vi "Simple UDP Test.vi"() -> ()   [LabVIEW 2016, in "instr.lvlib"]
doc: "Test VI using all other VIs.\nThis should help you to gest startet with your application."
uses:
  instr.lvlib
  IO State.ctl
  Digital Mode.ctl
panel:
  in  "local port":u16=61557
  in  "controllino ip":string="192.168.0.12"
  in  "controllino port":u16=8888
  in  "Send RAW":bool
  out "Memory Data Readback":i16
  in  "Memory Value":i16
  in  "Memory Addr":u16
  in  "Set Memory":bool
  in  "Set All Config":bool
  out "Digital Mode":T1[](array[typedef]) items=["Output"=79, "Input_Pullup"=80, "Input"=73]
  out "Inputs":bool[](array[boolean])
  out "dt (ms)":u32
  out "Analog Value":u16
  in  "Read Analog":bool
  out "Analog Values":u16[](array[numeric])
  in  "Analog Number":u16
  in  "Digital Mode":T1=73 items=["Output"=79, "Input_Pullup"=80, "Input"=73]
  in  "Set Config":bool
  in  "Set All Relay":bool
  in  "Set All Digital":bool
  in  "Digital State":T2 items=["LOW", "HIGH"]
  in  "Digital Number":u16
  in  "Relay State":T2 items=["LOW", "HIGH"]
  in  "Relay Number":u16
  in  "Set Digital":bool
  in  "Set Relay":bool
  out "Digitals":bool[](array[boolean])
  out "Relays":bool[](array[boolean])
  in  "stop":bool
  out "RAW Reply":string
  in  "RAW":string
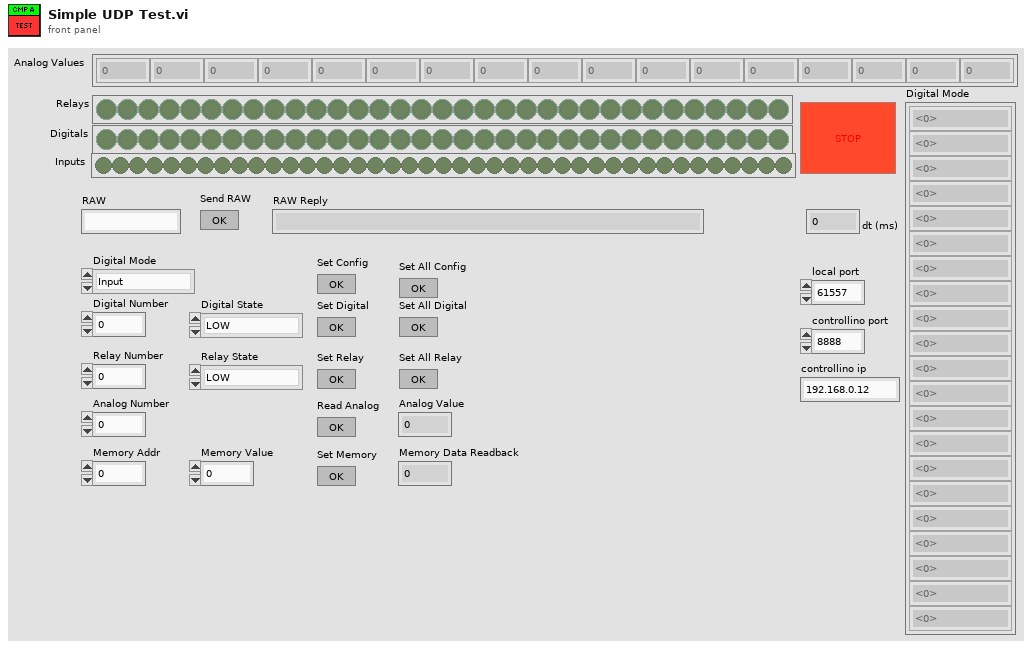
[diagram p1: front panel]
types:
  T1 = typedef "instr.lvlib/Digital Mode.ctl" = u16
  T2 = typedef "instr.lvlib/IO State.ctl" = u16
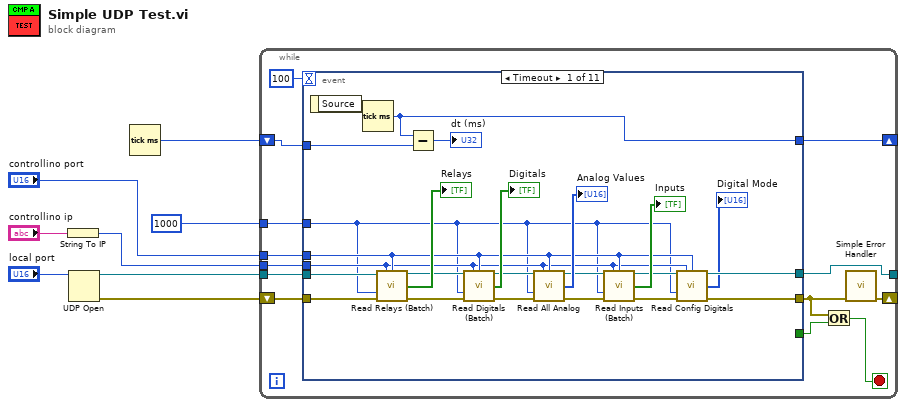
[diagram p0: block diagram]
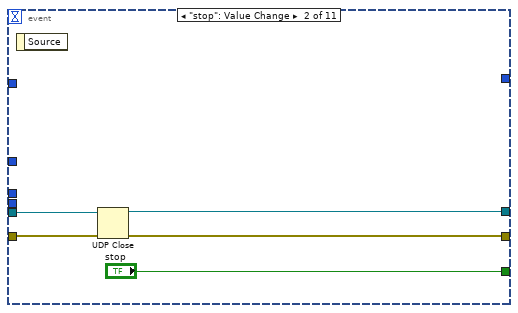
[diagram p2: hidden frame]
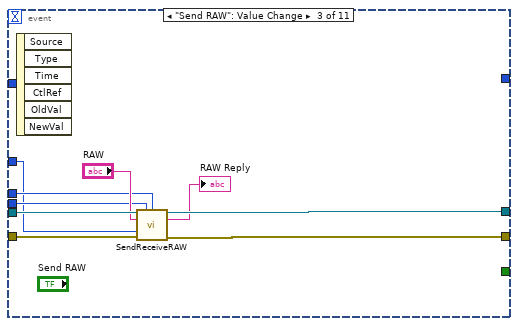
[diagram p3: hidden frame]
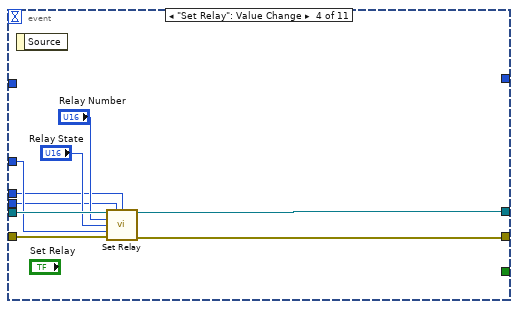
[diagram p4: hidden frame]
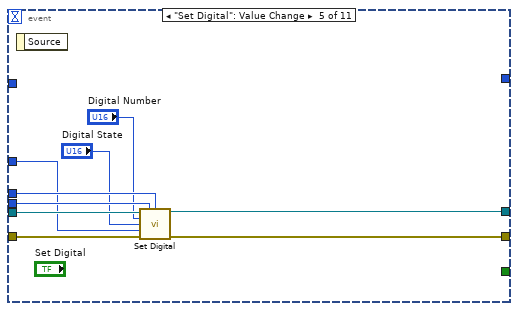
[diagram p5: hidden frame]
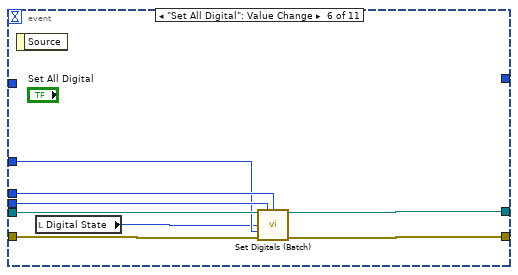
[diagram p6: hidden frame]
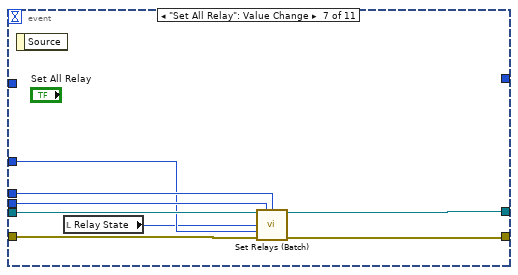
[diagram p7: hidden frame]
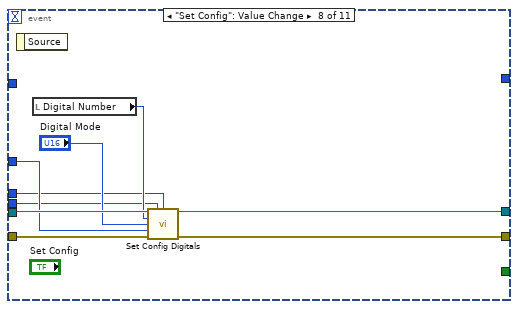
[diagram p8: hidden frame]
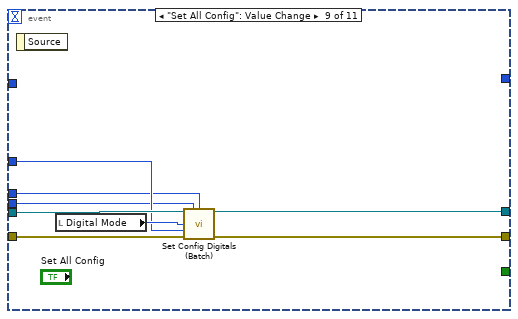
[diagram p9: hidden frame]
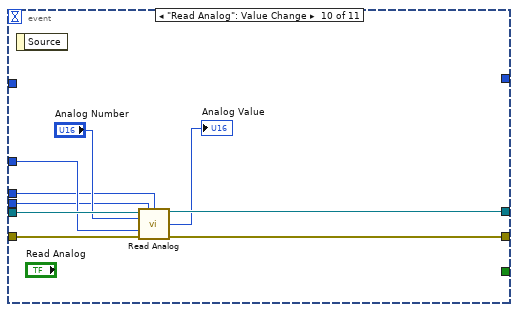
[diagram p10: hidden frame]
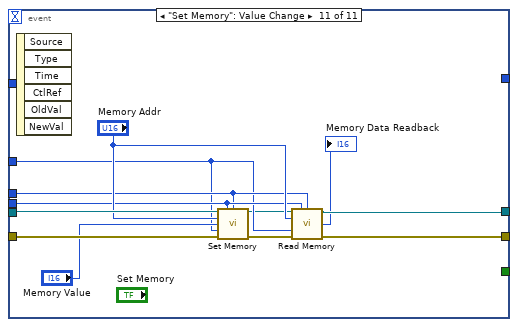
[diagram p11: hidden frame]
diagram:
  n1 = String To IP(1:"controllino ip") -> (0:w4:u32)
  n2 = UDP Open(11:"local port") -> (port=w6:refnum<k16>, 0:w5:errorcluster)  [unwired: 4 in, 1 out]
  n3 = Tick Count (ms)() -> (millisecond timer value=w1:u32)
  n4 = while {
    tunnel: w6 -> [w20]
    tunnel: [w18] -> _
    tunnel: w4 -> [w17]
    tunnel: "controllino port" -> [w16]
    tunnel: 1000 ("timeout ms (1000)") -> [w15]
    shift-right: [w14] -> _
    shift-left: w5 -> [w19]
    shift-right: [w12] -> _
    shift-left: w1 -> [w13]
    stop <- w9 stop-if-true
    n5 = event shown="[0] Timeout" {
      selector: _ -> [_ _ _ _ _ _ _ _ _ _ _]
      dyn-events: _ -> [_ _ _ _ _ _ _ _ _ _ _]
      timeout: 100 -> [_ _ _ _ _ _ _ _ _ _ _]
      tunnel: w20 -> [w44 w47 w54 w66 w74 w81 w92 w98 w107 w117 w129]
      tunnel: w19 -> [w43 w48 w58 w67 w76 w84 w91 w101 w108 w118 w130]
      tunnel: [w28 w46 w57 w64 w75 w83 w90 w100 w102 w112 w127] -> w11
      tunnel: [w27 w45 w56 w65 w73 w82 w89 w99 w103 w111 w121] -> w18
      tunnel: w17 -> [w24 _ w52 w60 w72 w79 w87 w93 w105 w113 w124]
      tunnel: w16 -> [w25 _ w51 w59 w71 w80 w88 w94 w104 w114 w123]
      tunnel: w15 -> [w23 _ w50 w62 w68 w78 w86 w95 w106 w115 w122]
      tunnel: [_ "stop" _ _ _ _ _ _ _ _ _] -> w10
      tunnel: w13 -> [w35 _ _ _ _ _ _ _ _ _ _]
      tunnel: [w34 _ _ _ _ _ _ _ _ _ _] -> w12
      event Timeout {
        n6 = event-data() -> ()  [unwired: 1 in, 1 out]
        n7 = Tick Count (ms)() -> (millisecond timer value=w34:u32)
        n8 = call "Read Relays (Batch).vi"("connection ID"=w44, "address"=w24, "port"=w25, "timeout ms (1000)"=w23, "error in (no error)"=w43) -> ("connection ID out"=w40:refnum<k16>, "Relays"=→"Relays":bool[], "error out"=w41:errorcluster)  [unwired: 7 in, 1 out]
        n9 = Subtract(x=w34, y=w35) -> (x-y=→"dt (ms)":u32)
        n10 = call "Read Digitals (Batch).vi"("connection ID"=w40, "address"=w24, "port"=w25, "timeout ms (1000)"=w23, "error in (no error)"=w41) -> ("connection ID out"=w38:refnum<k16>, "Digitals"=→"Digitals":bool[], "error out"=w37:errorcluster)  [unwired: 7 in, 1 out]
        n11 = call "Read All Analog.vi"("connection ID"=w38, "address"=w24, "port"=w25, "timeout ms (1000)"=w23, "error in (no error)"=w37) -> ("connection ID out"=w31:refnum<k16>, "Analog Values"=→"Analog Values":u16[], "error out"=w32:errorcluster)  [unwired: 7 in, 1 out]
        n12 = call "Read Inputs (Batch).vi"("connection ID"=w31, "address"=w24, "port"=w25, "timeout ms (1000)"=w23, "error in (no error)"=w32) -> ("connection ID out"=w26:refnum<k16>, "Inputs"=→"Inputs":bool[], "error out"=w29:errorcluster)  [unwired: 7 in, 1 out]
        n13 = call "Read Config Digitals.vi"("connection ID"=w26, "address"=w24, "port"=w25, "timeout ms (1000)"=w23, "error in (no error)"=w29) -> ("connection ID out"=w27:refnum<k16>, "Digital Mode"=→"Digital Mode":T1[], "error out"=w28:errorcluster)  [unwired: 7 in, 1 out]
      }
      event "stop": Value Change {
        n14 = event-data() -> ()  [unwired: 1 in, 1 out]
        n15 = UDP Close(connection ID=w47, 8:w48) -> (connection ID out=w45:refnum<k16>, error out=w46:errorcluster)
      }
      event "Send RAW": Value Change {
        n16 = event-data() -> ()  [unwired: 1 in, 6 out]
        n17 = call "SendReceiveRAW.vi"("connection ID"=w54, "address"=w52, "port"=w51, "RAW data in"="RAW", "timeout ms (1000)"=w50, "error in (no error)"=w58) -> ("connection ID out"=w56:refnum<k16>, "received data"=→"RAW Reply":string, "error out"=w57:errorcluster)  [unwired: 7 in]
      }
      event "Set Relay": Value Change {
        n18 = event-data() -> ()  [unwired: 1 in, 1 out]
        n19 = call "Set Relay.vi"("connection ID"=w66, "address"=w60, "port"=w59, "Relay Number"="Relay Number", "Relay State"="Relay State", "timeout ms (1000)"=w62, "error in (no error)"=w67) -> ("connection ID out"=w65:refnum<k16>, "error out"=w64:errorcluster)  [unwired: 6 in, 1 out]
      }
      event "Set Digital": Value Change {
        n20 = event-data() -> ()  [unwired: 1 in, 1 out]
        n21 = call "Set Digital.vi"("connection ID"=w74, "address"=w72, "port"=w71, "Digital Number"="Digital Number", "Digital State"="Digital State", "timeout ms (1000)"=w68, "error in (no error)"=w76) -> ("connection ID out"=w73:refnum<k16>, "error out"=w75:errorcluster)  [unwired: 6 in, 1 out]
      }
      event "Set All Digital": Value Change {
        n22 = event-data() -> ()  [unwired: 1 in, 1 out]
        n23 = local read "Digital State"() -> (w77:T2)
        n24 = call "Set Digitals (Batch).vi"("connection ID"=w81, "address"=w79, "port"=w80, "Digital State"=w77, "timeout ms (1000)"=w78, "error in (no error)"=w84) -> ("connection ID out"=w82:refnum<k16>, "error out"=w83:errorcluster)  [unwired: 7 in, 1 out]
      }
      event "Set All Relay": Value Change {
        n25 = event-data() -> ()  [unwired: 1 in, 1 out]
        n26 = local read "Relay State"() -> (w85:T2)
        n27 = call "Set Relays (Batch).vi"("connection ID"=w92, "address"=w87, "port"=w88, "Relay State"=w85, "timeout ms (1000)"=w86, "error in (no error)"=w91) -> ("connection ID out"=w89:refnum<k16>, "error out"=w90:errorcluster)  [unwired: 7 in, 1 out]
      }
      event "Set Config": Value Change {
        n28 = event-data() -> ()  [unwired: 1 in, 1 out]
        n29 = local read "Digital Number"() -> (w97:u16)
        n30 = call "Set Config Digitals.vi"("connection ID"=w98, "address"=w93, "port"=w94, "Digital Number"=w97, "Digital Mode"="Digital Mode", "timeout ms (1000)"=w95, "error in (no error)"=w101) -> ("connection ID out"=w99:refnum<k16>, "error out"=w100:errorcluster)  [unwired: 6 in, 1 out]
      }
      event "Set All Config": Value Change {
        n31 = event-data() -> ()  [unwired: 1 in, 1 out]
        n32 = local read "Digital Mode"() -> (w109:T1)
        n33 = call "Set Config Digitals (Batch).vi"("connection ID"=w107, "address"=w105, "port"=w104, "Digital Mode"=w109, "timeout ms (1000)"=w106, "error in (no error)"=w108) -> ("connection ID out"=w103:refnum<k16>, "error out"=w102:errorcluster)  [unwired: 7 in, 1 out]
      }
      event "Read Analog": Value Change {
        n34 = event-data() -> ()  [unwired: 1 in, 1 out]
        n35 = call "Read Analog.vi"("connection ID"=w117, "address"=w113, "port"=w114, "Analog Number"="Analog Number", "timeout ms (1000)"=w115, "error in (no error)"=w118) -> ("connection ID out"=w111:refnum<k16>, "Analog Value"=→"Analog Value":u16, "error out"=w112:errorcluster)  [unwired: 6 in, 1 out]
      }
      event "Set Memory": Value Change {
        n36 = event-data() -> ()  [unwired: 1 in, 6 out]
        n37 = call "Set Memory.vi"("connection ID"=w129, "address"=w124, "port"=w123, "Digital Number"="Memory Addr", "Data"="Memory Value", "timeout ms (1000)"=w122, "error in (no error)"=w130) -> ("connection ID out"=w119:refnum<k16>, "error out"=w126:errorcluster)  [unwired: 6 in, 1 out]
        n38 = call "Read Memory.vi"("connection ID"=w119, "address"=w124, "port"=w123, "Memory Address"="Memory Addr", "timeout ms (1000)"=w122, "error in (no error)"=w126) -> ("connection ID out"=w121:refnum<k16>, "Memory Data"=→"Memory Data Readback":i16, "error out"=w127:errorcluster)  [unwired: 6 in, 1 out]
      }
    }
    n39 = Or(x=w11, y=w10) -> (x .or. y?=w9:bool)
    n40 = call <vilib>:"Simple Error Handler.vi"("error in (no error)"=w11) -> ("error out"=w14:errorcluster)  [unwired: 4 in, 4 out]
  }
